vi "Teleop.vi"(10 "Match Info":T2={"Autonomous Elapsed Seconds"=0.0, "TeleOp Elapsed Seconds"=0.0, "Disabled Elapsed Seconds"=0.0, "Visited Autonomous"=FALSE, "Visited TeleOp"=FALSE, "Visited Disabled"=FALSE, "Autonomous Settings"={"Autonomous Style"=enum."Independent", "VI Refnum"=refnum}}, 11 "Call Context":T3) -> ()   [LabVIEW 2019]
doc: "This VI is called for each enabled TeleOp packet received from the DS. It is typically used to read from joysticks and other inputs and update I/O or setpoints for timed control loops. It should complete and return within 20 milliseconds or risk missing DS packets."
uses:
  <vilib>/Rock Robotics/WPI/DriverStation/WPI_DriverStationDerivedRobotMode.ctl
  <vilib>/Rock Robotics/WPI/DriverStation/WPI_DriverStationMatch Info.ctl
  <vilib>/Rock Robotics/WPI/Utilities/WPI_GetSetVariantRefNum.vi
  <vilib>/Rock Robotics/Network Tables/NT Write Boolean Array.vi
  <vilib>/Rock Robotics/Network Tables/NT Write Numeric Array.vi
panel:
  in  "Two Controller\nFeed axis?":bool
  in  "Two controller\nFeed axis":dbl
  in  "Feed button":dbl=5.0
  in  "Feed one control":bool=TRUE
  in  "feeder multiplier":dbl(slide)=1.0 scale=0.0..1.0
  in  "Two Controller\nshooter axis?":bool
  in  "Two controller\nShooter axis":dbl
  in  "Shoot button":dbl=4.0
  in  "One contoller":bool=TRUE
  in  "shoot multiplier":dbl(slide)=1.0 scale=0.0..1.0
  in  "speed multiplier":dbl(slide)=1.0 scale=0.0..1.0
  in  "Speed?":bool
  in  "Enum":T1(ring)=enum."One Controller Tank"
  in  "Controller 2 inverted":bool
  in  "Controller 2 Joystick":dbl min=0.0 max=6.0 step=1.0
  in  "Quickturn button":dbl min=0.0 max=12.0 step=1.0
  in  "Inverted One":bool
  in  "Inverted Two":bool
  in  "Joystick Two":dbl=5.0 min=0.0 max=6.0 step=1.0
  in  "Joystick One":dbl=1.0 min=0.0 max=6.0 step=1.0
  # "Drive"
  # "Multiplier"
  # "Shooter"
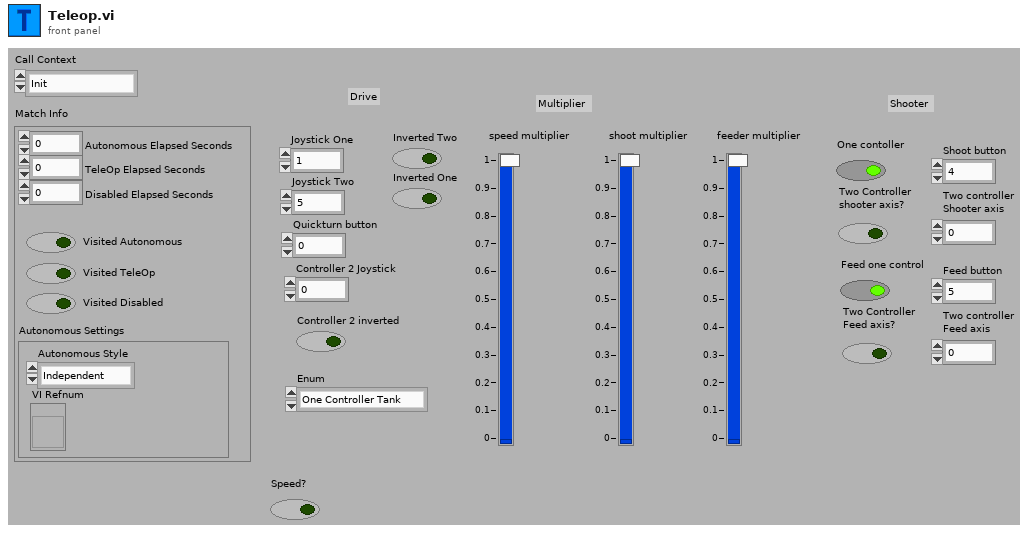
[diagram p1: front panel]
types:
  T1 = enum16{"Arcade", "One Controller Tank", "Two Controller Tank", "Cheesy Drive"}
  T2 = typedef "WPI_DriverStationMatch Info.ctl" = cluster{"Autonomous Elapsed Seconds":dbl, "TeleOp Elapsed Seconds":dbl, "Disabled Elapsed Seconds":dbl, "Visited Autonomous":bool, "Visited TeleOp":bool, "Visited Disabled":bool, "Autonomous Settings":cluster{"Autonomous Style":enum16{"Iterative", "Independent"}, "VI Refnum":refnum<vi>}}
  T3 = typedef "WPI_DriverStationDerivedRobotMode.ctl" = enum16{"Init", "Execute", "Stop"}
  T4 = enum16{"Arcade", "One Joystick Tank", "Two Joystick Tank", "Cheesy Drive", ""}
  T5 = typedef "WPI_JoystickDevRef.ctl" = cluster{"Device":T6}
  T6 = typedef "WPI_JoystickDeviceEnum.ctl" = enum16{"USB 0", "USB 1", "USB 2", "USB 3", "USB 4", "USB 5"}
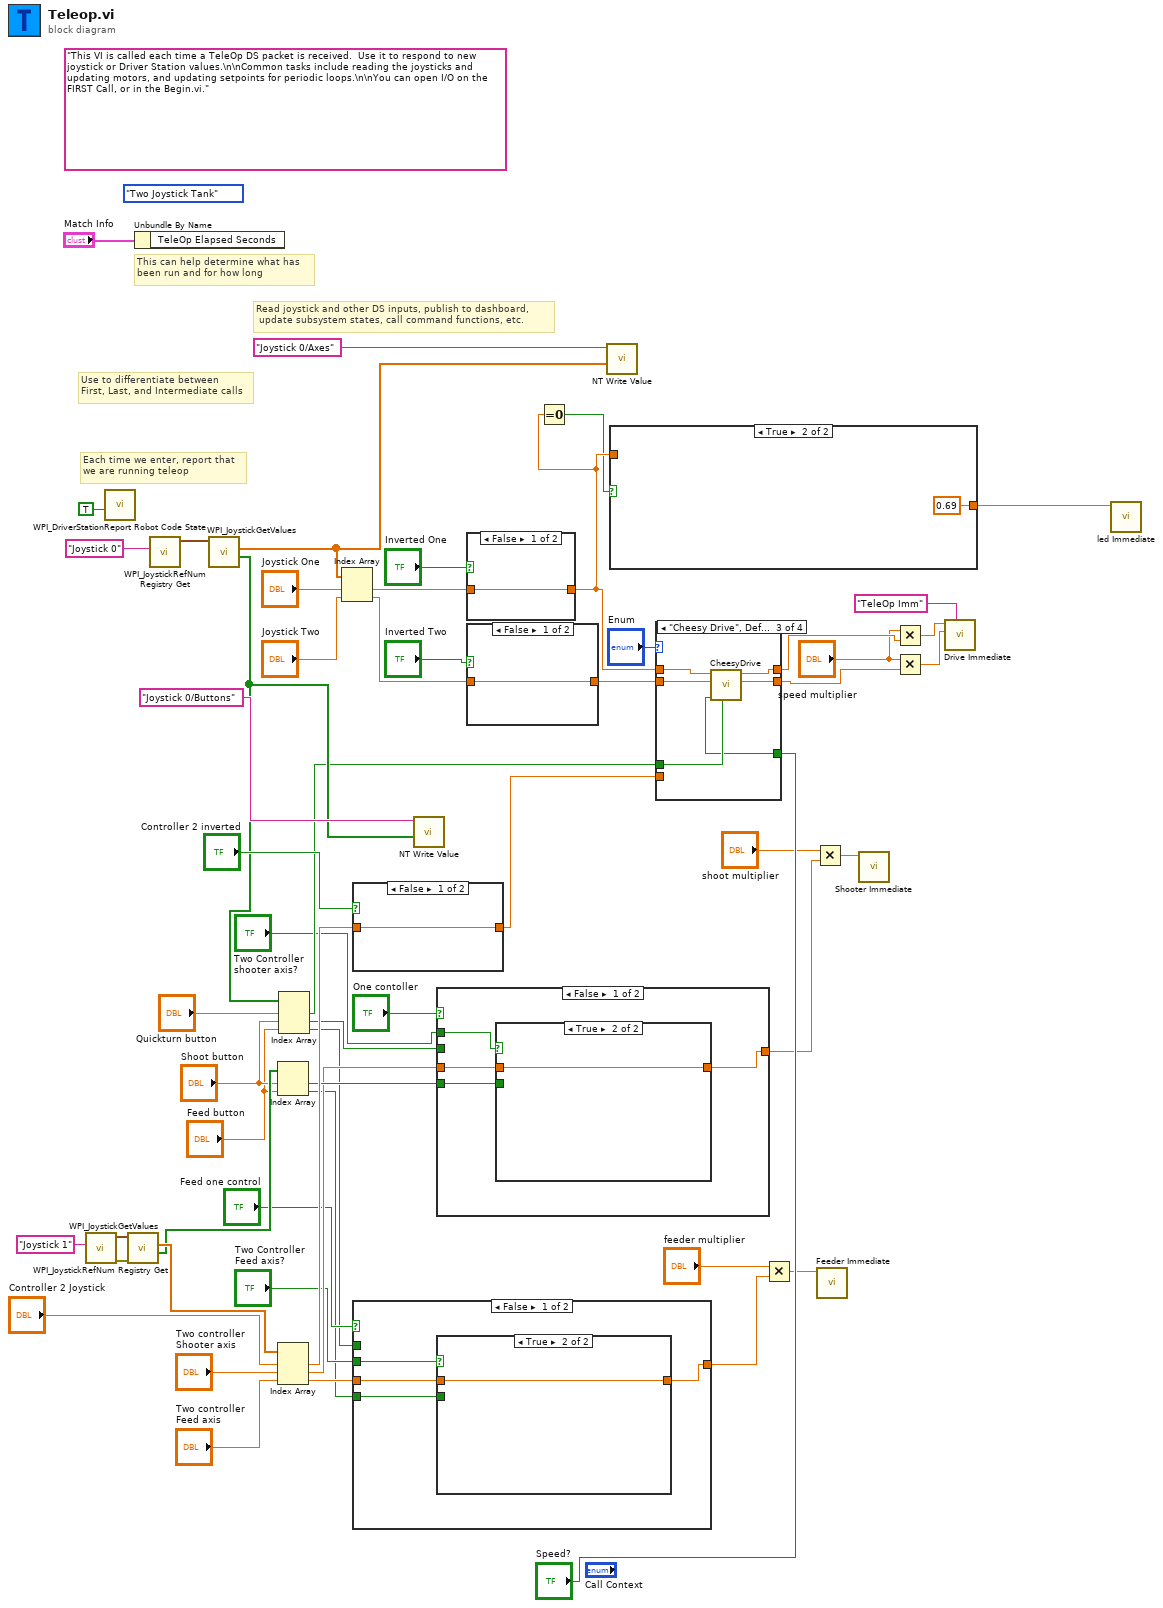
[diagram p0: block diagram]
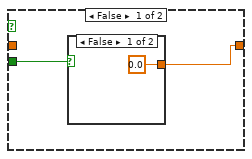
[diagram p2: hidden frame]
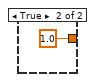
[diagram p3: hidden frame]
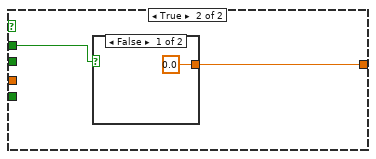
[diagram p4: hidden frame]
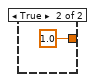
[diagram p5: hidden frame]
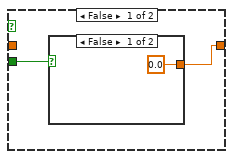
[diagram p6: hidden frame]
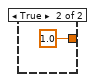
[diagram p7: hidden frame]
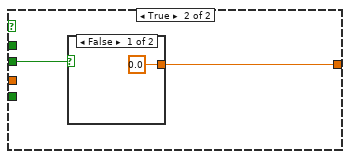
[diagram p8: hidden frame]
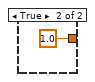
[diagram p9: hidden frame]
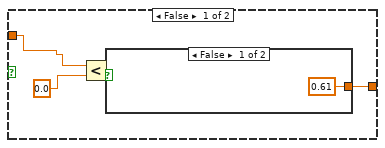
[diagram p10: hidden frame]
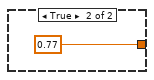
[diagram p11: hidden frame]
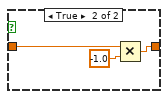
[diagram p12: hidden frame]
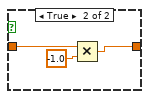
[diagram p13: hidden frame]
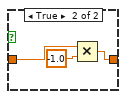
[diagram p14: hidden frame]
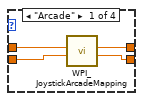
[diagram p15: hidden frame]
diagram:
  (unwired) T4."Two Joystick Tank"
  (unwired) "This VI is called each time a TeleOp DS packet is received.  Use it to respond to new joystick or Driver Station values.\n\nCommon tasks include reading the joysticks and updating motors, and updating setpoints for periodic loops.\n\nYou can open I/O on the FIRST Call, or in the Begin.vi."
  # "Read joystick and other DS inputs, publish to dashboard,\n update subsystem states, call command functions, etc."
  # "Each time we enter, report that\nwe are running teleop"
  # "Use to differentiate between\nFirst, Last, and Intermediate calls"
  # "This can help determine what has\nbeen run and for how long"
  n1 = call <vilib>:"WPI_JoystickRefNum Registry Get.vi"("refnum name"="Joystick 1") -> ("error out"=w40:errorcluster, "JoystickDevRef"=w41:T5)  [unwired: 1 in, 8 out]
  n2 = call <vilib>:"WPI_DriverStationReport Robot Code State.vi"("TeleOp"=TRUE ("Autonomous")) -> ()  [unwired: 10 in, 1 out]
  n3 = call <vilib>:"WPI_JoystickGetValues.vi"("error in (no error)"=w40, "JoystickDevRef"=w41) -> ("Buttons"=w19:bool[], "Axes"=w38:dbl[])  [unwired: 5 in, 3 out]
  n4 = Unbundle By Name("Match Info") -> ()  [unwired: 1 out]
  n5 = call <vilib>:"WPI_JoystickRefNum Registry Get.vi"("refnum name"="Joystick 0") -> ("JoystickDevRef"=w54:T5)  [unwired: 1 in, 9 out]
  n6 = call <vilib>:"WPI_JoystickGetValues.vi"("JoystickDevRef"=w54) -> ("Buttons"=w33:bool[], "Axes"=w51:dbl[])  [unwired: 6 in, 3 out]
  n7 = Index Array(array=w19, index #1="Shoot button", index #2="Feed button") -> (element #1=w18:bool, element #2=w2:bool)
  n8 = Index Array(array=w38, index #1="Controller 2 Joystick", index #2="Two controller\nShooter axis", index #3="Two controller\nFeed axis") -> (element #1=w35:dbl, element #2=w11:dbl, element #3=w5:dbl)
  n9 = Index Array(array=w33, index #1="Quickturn button", index #2="Shoot button", index #3="Feed button") -> (element #1=w31:bool, element #2=w20:bool, element #3=w1:bool)
  n10 = Index Array(array=w51, index #1="Joystick One", index #2="Joystick Two") -> (element #1=w45:dbl, element #2=w44:dbl)
  n11 = case shown="False" "Controller 2 inverted" {
    tunnel: w35 -> [w58 w60]
    tunnel: [w58 w59] -> w34
    frame False {
    }
    frame True {
      n12 = Multiply(x=w60, y=-1.0) -> (x*y=w59:dbl)
    }
  }
  n13 = case shown="False" "Feed one control" {
    tunnel: w1 -> [_ w72]
    tunnel: w2 -> [w65 _]
    tunnel: [w64 w71] -> w9
    tunnel: "Two Controller\nFeed axis?" -> [w63 _]
    tunnel: w5 -> [w62 _]
    frame False {
      n14 = case shown="True" w63 {
        tunnel: w65 -> [w67 _]
        tunnel: [w66 w70] -> w64
        tunnel: w62 -> [_ w70]
        frame False {
          n15 = case shown="False" w67 {
            tunnel: [0.0 1.0] -> w66
            frame False {
            }
            frame True {
            }
          }
        }
        frame True {
        }
      }
    }
    frame True {
      n16 = case shown="False" w72 {
        tunnel: [0.0 1.0] -> w71
        frame False {
        }
        frame True {
        }
      }
    }
  }
  n17 = call-poly <vilib>:"NT Write Value.vi"("Boolean Array"=w33, "Name"="Joystick 0/Buttons") -> ()  [unwired: 9 in, 1 out]
  n18 = case shown="False" "One contoller" {
    tunnel: w20 -> [_ w85]
    tunnel: w18 -> [w78 _]
    tunnel: [w77 w84] -> w15
    tunnel: "Two Controller\nshooter axis?" -> [w76 _]
    tunnel: w11 -> [w75 _]
    frame False {
      n19 = case shown="True" w76 {
        tunnel: w78 -> [w80 _]
        tunnel: [w79 w83] -> w77
        tunnel: w75 -> [_ w83]
        frame False {
          n20 = case shown="False" w80 {
            tunnel: [0.0 1.0] -> w79
            frame False {
            }
            frame True {
            }
          }
        }
        frame True {
        }
      }
    }
    frame True {
      n21 = case shown="False" w85 {
        tunnel: [0.0 1.0] -> w84
        frame False {
        }
        frame True {
        }
      }
    }
  }
  n22 = case shown="False" "Inverted One" {
    tunnel: w45 -> [w88 w90]
    tunnel: [w88 w89] -> w29
    frame False {
    }
    frame True {
      n23 = Multiply(x=w90, y=-1.0) -> (x*y=w89:dbl)
    }
  }
  n24 = case shown="False" "Inverted Two" {
    tunnel: w44 -> [w92 w94]
    tunnel: [w92 w93] -> w43
    frame False {
    }
    frame True {
      n25 = Multiply(x=w94, y=-1.0) -> (x*y=w93:dbl)
    }
  }
  n26 = Equal To 0?(x=w29) -> (x = 0?=w28:bool)
  n27 = call-poly <vilib>:"NT Write Value.vi"("Numeric Array"=w51, "Name"="Joystick 0/Axes") -> ()  [unwired: 9 in, 1 out]
  n28 = case shown="True" w28 {
    tunnel: [w97 0.69] -> w30
    tunnel: w29 -> [w96 _]
    frame False {
      n29 = Less?(x=w96, y=0.0) -> (x < y?=w99:bool)
      n30 = case shown="False" w99 {
        tunnel: [0.61 0.77] -> w97
        frame False {
        }
        frame True {
        }
      }
    }
    frame True {
    }
  }
  n31 = case shown="\"Cheesy Drive\", Default" "Enum" {
    tunnel: w29 -> [w106 w108 w114 w116]
    tunnel: w43 -> [w105 _ w113 w115]
    tunnel: [w104 w108 w111 w116] -> w26
    tunnel: [w103 w107 w110 w115] -> w24
    tunnel: w34 -> [_ w107 _ _]
    tunnel: w31 -> [_ _ w112 _]
    tunnel: "Speed?" -> [_ _ w109 _]
    frame "Arcade" {
      n32 = call <vilib>:"WPI_JoystickArcadeMapping.vi"("Y axis value"=w105, "X axis value"=w106) -> ("Right Motor Value"=w103:dbl, "Left Motor Value"=w104:dbl)  [unwired: 8 in]
    }
    frame "Two Controller Tank" {
    }
    frame "Cheesy Drive", Default {
      n33 = call "CheesyDrive.vi"("Quickturn"=w112, "Fast Mode"=w109, "Wheel"=w113, "Throttle"=w114) -> ("Right PWM"=w110:dbl, "Left PWM"=w111:dbl)  [unwired: 6 in]
    }
    frame "One Controller Tank" {
    }
  }
  n34 = Multiply(x="feeder multiplier", y=w9) -> (x*y=w10:dbl)
  n35 = Multiply(x="shoot multiplier", y=w15) -> (x*y=w16:dbl)
  n36 = call "Feeder Immediate.vi"("Setpoint"=w10) -> ()  [unwired: 10 in, 1 out]
  n37 = call "Shooter Immediate.vi"("Setpoint"=w16) -> ()  [unwired: 10 in, 1 out]
  n38 = Multiply(x="speed multiplier", y=w26) -> (x*y=w25:dbl)
  n39 = Multiply(x="speed multiplier", y=w24) -> (x*y=w22:dbl)
  n40 = call "Drive Immediate.vi"("Description"="TeleOp Imm", "Right Setpoint"=w22, "Left Setpoint"=w25) -> ()  [unwired: 8 in, 1 out]
  n41 = call "led Immediate.vi"("Setpoint"=w30) -> ()  [unwired: 10 in, 1 out]
